vi "SearchVirtualFolder.vi"(8 "error in (no error)":errorcluster, 10 "Actor Method VI Name":string, 11 "ProjectItemIn":refnum<vi>) -> (0 "error out":errorcluster, 1 "Found?":bool, 2 "SubFolder":string)   [LabVIEW 2015, in "CS++Actor.lvlib" / "CS++Actor.lvclass"]
uses:
  CS++Actor.lvclass
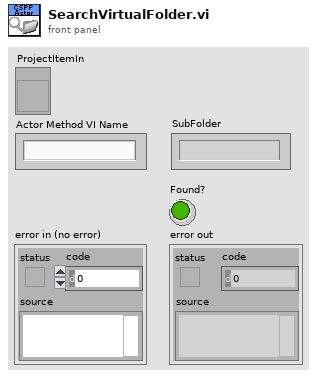
[diagram p1: front panel]
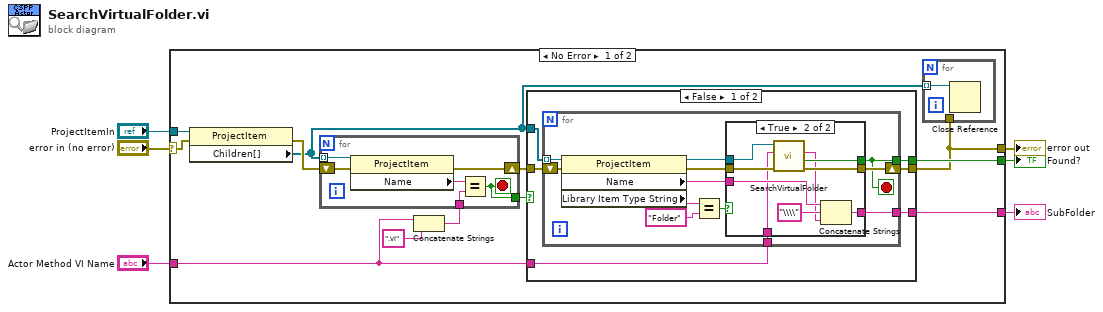
[diagram p0: block diagram]
diagram:
  n1 = case shown="No Error" "error in (no error)" {
    selector: "error in (no error)" -> [w11 w56]
    tunnel: "ProjectItemIn" -> [w12 _]
    tunnel: "Actor Method VI Name" -> [w7 _]
    tunnel: [w16 _] -> w4
    tunnel: [w15 _] -> w3
    tunnel: [w8 w56] -> w1
    frame No Error {
      n2 = property class="ProjectItem"(reference=w12, error in=w11) -> (error out=w10:errorcluster, "Children[]"=w9:refnum<vi>[])  [unwired: 1 out]
      n3 = Concatenate Strings(w7, ".vi" ("string")) -> (w13:string)
      n4 = for {
        tunnel: w9 -> [w55] mode=indexing
        tunnel: w13 -> [w53]
        tunnel: [w52] -> w18
        shift-right: [w50] -> w17
        shift-left: w10 -> [w51]
        stop <- w52 stop-if-true
        n5 = property class="ProjectItem"(reference=w55, error in=w51) -> (error out=w50:errorcluster, "Name"=w54:string)  [unwired: 1 out]
        n6 = Equal?(x=w54, y=w53) -> (x = y?=w52:bool)
      }
      n7 = case shown="False" w18 {
        selector: w18 -> [_ w49]
        tunnel: w17 -> [w20 w48]
        tunnel: [w25 w49] -> w16
        tunnel: [w24 _] -> w15
        tunnel: w7 -> [w23 _]
        tunnel: [w22 w48] -> w8
        tunnel: w9 -> [w21 _]
        frame False {
          n8 = for {
            tunnel: w21 -> [w35] mode=indexing
            shift-right: [w37] -> w22
            shift-left: w20 -> [w33]
            tunnel: [w36] -> w25
            tunnel: [w31] -> w24
            tunnel: w23 -> [w29]
            stop <- w36 stop-if-true
            n9 = property class="ProjectItem"(reference=w35, error in=w33) -> (reference out=w34:refnum<vi>, error out=w32:errorcluster, "Name"=w30:string, "Library Item Type String"=w27:string)
            n10 = Equal?(x=w27, y="Folder" ("Type")) -> (x = y?=w26:bool)
            n11 = case shown="True" w26 {
              tunnel: [w38 w47] -> w37
              tunnel: [_ w46] -> w36
              tunnel: w34 -> [_ w45]
              tunnel: w32 -> [w38 w44]
              tunnel: [_ w42] -> w31
              tunnel: w30 -> [_ w41]
              tunnel: w29 -> [_ w39]
              frame False {
              }
              frame True {
                n12 = call "SearchVirtualFolder.vi"("error in (no error)"=w44, "Actor Method VI Name"=w39, "ProjectItemIn"=w45) -> ("error out"=w47:errorcluster, "Found?"=w46:bool, "SubFolder"=w40:string)  [unwired: 6 in]
                n13 = Concatenate Strings(w41, "\\\\" ("string"), w40) -> (w42:string)
              }
            }
          }
        }
        frame True {
        }
      }
      n14 = for {
        tunnel: w9 -> [w19] mode=indexing
        tunnel: w8 -> [_]
        n15 = Close Reference(reference=w19) -> ()  [unwired: 1 in, 1 out]
      }
    }
    frame Error {
    }
  }
  "error out" <- w1
  "SubFolder" <- w3
  "Found?" <- w4
